vi "Player Info.vi"(11 "Protector in":refnum<class "Protector.lvclass">) -> (1 "Victory Speech":string, 2 "Name":string, 3 "Protector out":refnum<class "Protector.lvclass">)   [LabVIEW 2015, in "Protector.lvclass"]
uses:
  Protector.lvclass
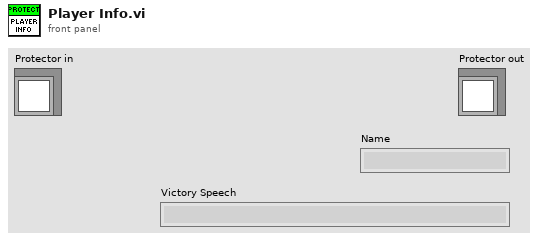
[diagram p1: front panel]
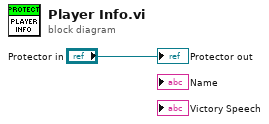
[diagram p0: block diagram]
diagram:
  "Protector out" <- "Protector in"
